vi "P3060_LoadFPGA.vi"(8 "错误输入":errorcluster caption="错误输入（无错误）", 10 "Bit文件路径":path, 11 "句柄输入":i32) -> (0 "错误输出":errorcluster, 2 "返回值":i32, 3 "句柄输出":i32)   [LabVIEW 2012]
doc: "发送异步通道数据"
uses:
  _SubVI/dll/P3060.dll
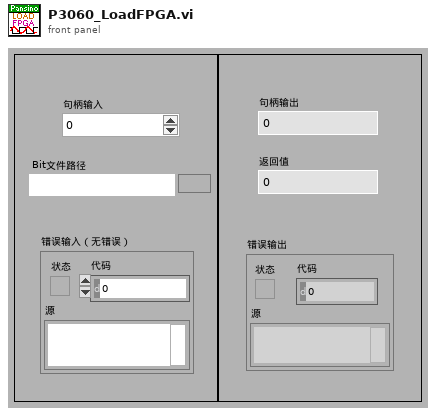
[diagram p1: front panel]
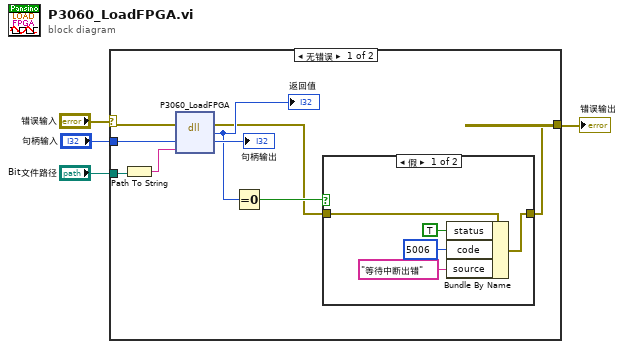
[diagram p0: block diagram]
diagram:
  n1 = case shown="无错误" "错误输入" {
    selector: "错误输入" -> [w13 w20]
    tunnel: [w7 w20] -> w3
    tunnel: "句柄输入" -> [w11 _]
    tunnel: "Bit文件路径" -> [w6 _]
    frame No Error {
      n2 = Path To String(path=w6) -> (string=w5:string)
      n3 = dll-call lib="C:/PLC_simulation/2014.3.10PLC_NEW/PLC_NEW/P3060NEW/_SubVI/dll/P3060.dll" fn="P3060_LoadFPGA"(error in=w13, "hDev"=w11, "Interval"=w5) -> (error out=w8:errorcluster, "return"=w10:i32, "hDev"=→"句柄输出":i32)  [unwired: 3 in, 1 out]
      "返回值" <- w10
      n4 = Equal To 0?(x=w10) -> (x = 0?=w9:bool)
      n5 = case shown="假" w9 {
        tunnel: [w17 w19] -> w7
        tunnel: w8 -> [w18 w19]
        frame False {
          n6 = Bundle By Name(cluster=w18, "status"=TRUE, "code"=5006, "source"="等待中断出错") -> (w17:errorcluster)
        }
        frame True {
        }
      }
    }
    frame Error {
    }
  }
  "错误输出" <- w3
